vi "Sig-Ana.vi"() -> ()   [LabVIEW 2022 SP3]
panel:
  out "Signalgraph":dynamicdata(graph) caption="Signalverlaufsgraph"
  in  "Stopp":bool
  out "Warnung Ueff > 5V":bool
  out "Effektiv Wert [Ueff]":dbl(slide) scale=0.0..15.0
  out "Spitze-Sptze Wert [Uss]":dbl(knob) scale=0.0..30.0
  out "Mittelwert  [U]":dbl(knob) scale=0.0..10.0
  in  "Amplitude Rechteck Signal [V]":dbl(slide) min=0.0 max=5.0 step=0.25 scale=0.0..5.0 scale format="%#.0f"
  in  "Amplitude Sinus Signal [V]":dbl(slide) min=0.0 max=10.0 step=0.5 scale=0.0..10.0 scale format="%#.1g"
  in  "Frequenz Rechteck Signal [Hz]":dbl(slide) min=0.0 max=250.0 step=1.0 scale=0.0..250.0 scale format="%#.0f"
  in  "Frequenz Sinus Signal [Hz]":dbl(slide) min=0.0 max=20.0 step=0.5 scale=0.0..20.0 scale format="%#.1g"
  # "Eingabefelder"
  # "Ausgabefelder"
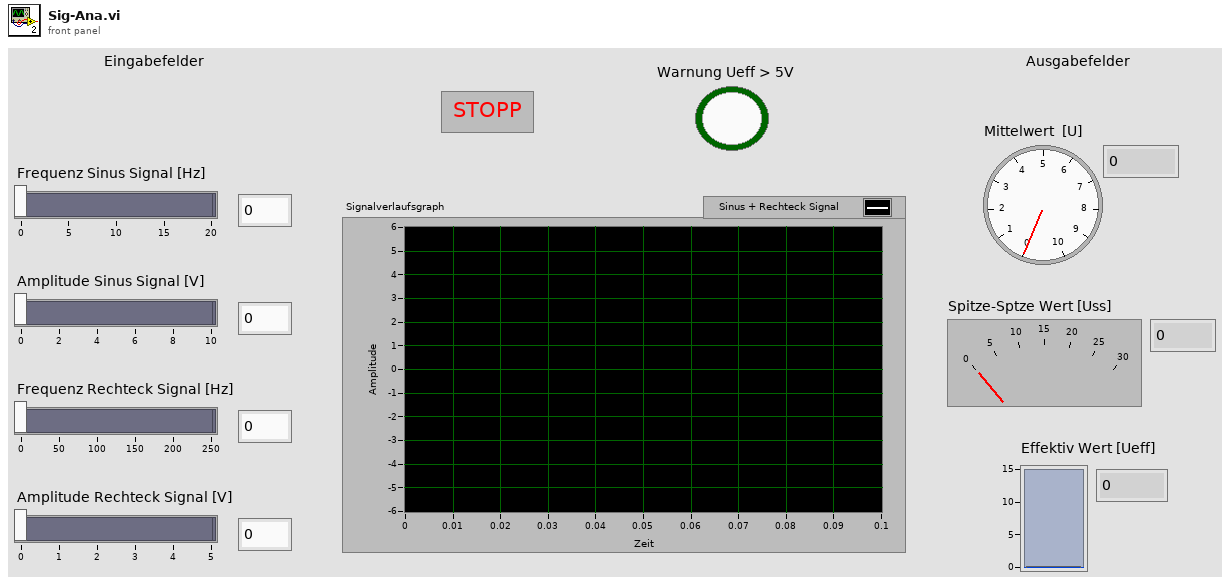
[diagram p1: front panel]
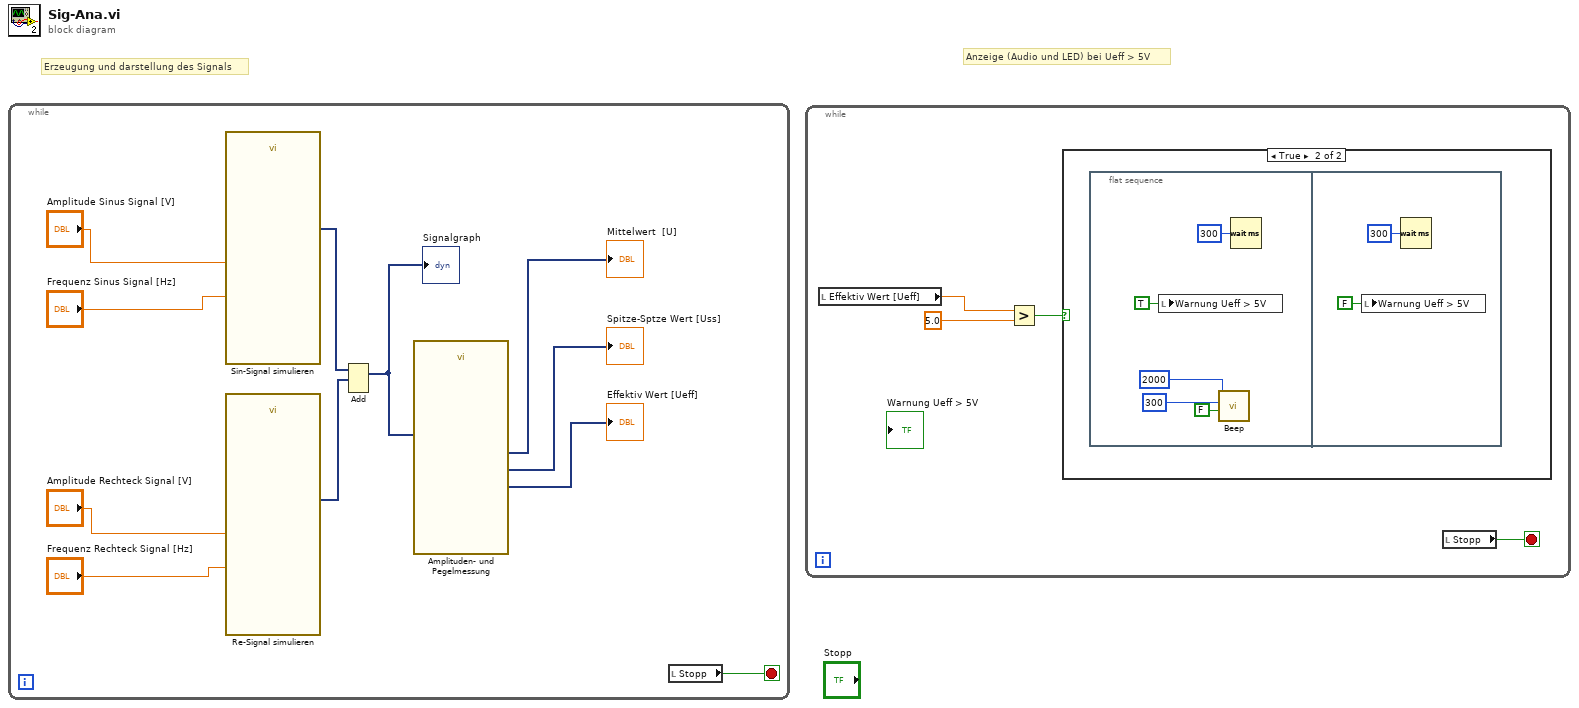
[diagram p0: block diagram]
diagram:
  # "Anzeige (Audio und LED) bei Ueff > 5V"
  # "Erzeugung und darstellung des Signals"
  n1 = while {
    stop <- w2 stop-if-true
    n2 = call "Sin-Signal simulieren"("Frequency"="Frequenz Sinus Signal [Hz]", "Amplitude"="Amplitude Sinus Signal [V]") -> ("Sinus"=w7:dynamicdata)  [unwired: 12 in, 1 out]
    n3 = call "Re-Signal simulieren"("Frequency"="Frequenz Rechteck Signal [Hz]", "Amplitude"="Amplitude Rechteck Signal [V]") -> ("Rechteck"=w6:dynamicdata)  [unwired: 12 in, 1 out]
    n4 = Add(1:w6, 2:w7) -> (0:w3:dynamicdata)  [unwired: 1 in, 1 out]
    "Signalgraph" <- w3
    n5 = call "Amplituden- und Pegelmessung"("Signals"=w3) -> ("Mean (DC)"=→"Mittelwert  [U]":dynamicdata, "RMS"=→"Effektiv Wert [Ueff]":dynamicdata, "Peak to Peak"=→"Spitze-Sptze Wert [Uss]":dynamicdata)  [unwired: 11 in, 1 out]
    n6 = local read "Stopp"() -> (w2:bool)
  }
  n7 = while {
    stop <- w15 stop-if-true
    n8 = local read "Effektiv Wert [Ueff]"() -> (w13:dbl)
    n9 = Greater?(x=w13, y=5.0) -> (0:w12:bool)
    n10 = case shown="True" w12 {
      frame False {
      }
      frame True {
        n11 = flat-sequence {
          frame #0 {
            n12 = local write "Warnung Ueff > 5V"(TRUE ("Warnung Ueff > 5V")) -> ()
            n13 = call <vilib>:"Beep.vi"("use system alert? (T)"=FALSE, "duration (msec)"=u32 300, "frequency (Hz)"=u32 2000) -> ()  [unwired: 9 in]
            n14 = Wait (ms)(milliseconds to wait=u32 300 ("Zu wartende ms")) -> ()  [unwired: 1 out]
          }
          frame #1 {
            n15 = local write "Warnung Ueff > 5V"(FALSE ("Warnung Ueff > 5V")) -> ()
            n16 = Wait (ms)(milliseconds to wait=u32 300 ("Zu wartende ms")) -> ()  [unwired: 1 out]
          }
        }
      }
    }
    n17 = local read "Stopp"() -> (w15:bool)
  }
